vi "StitchTest.vi"() -> ()   [LabVIEW 2014]
uses:
  <vilib>/picture/picture.llb/imagedata.ctl
panel:
  in  "SaveJPEG":bool
  out "Intensity Graph":u8[][](graph)
  out "Yind":i32[](array[numeric])
  out "Xind":i32[](array[numeric])
  out "filenames":string[](array[string])
  in  "PathToVK4":path
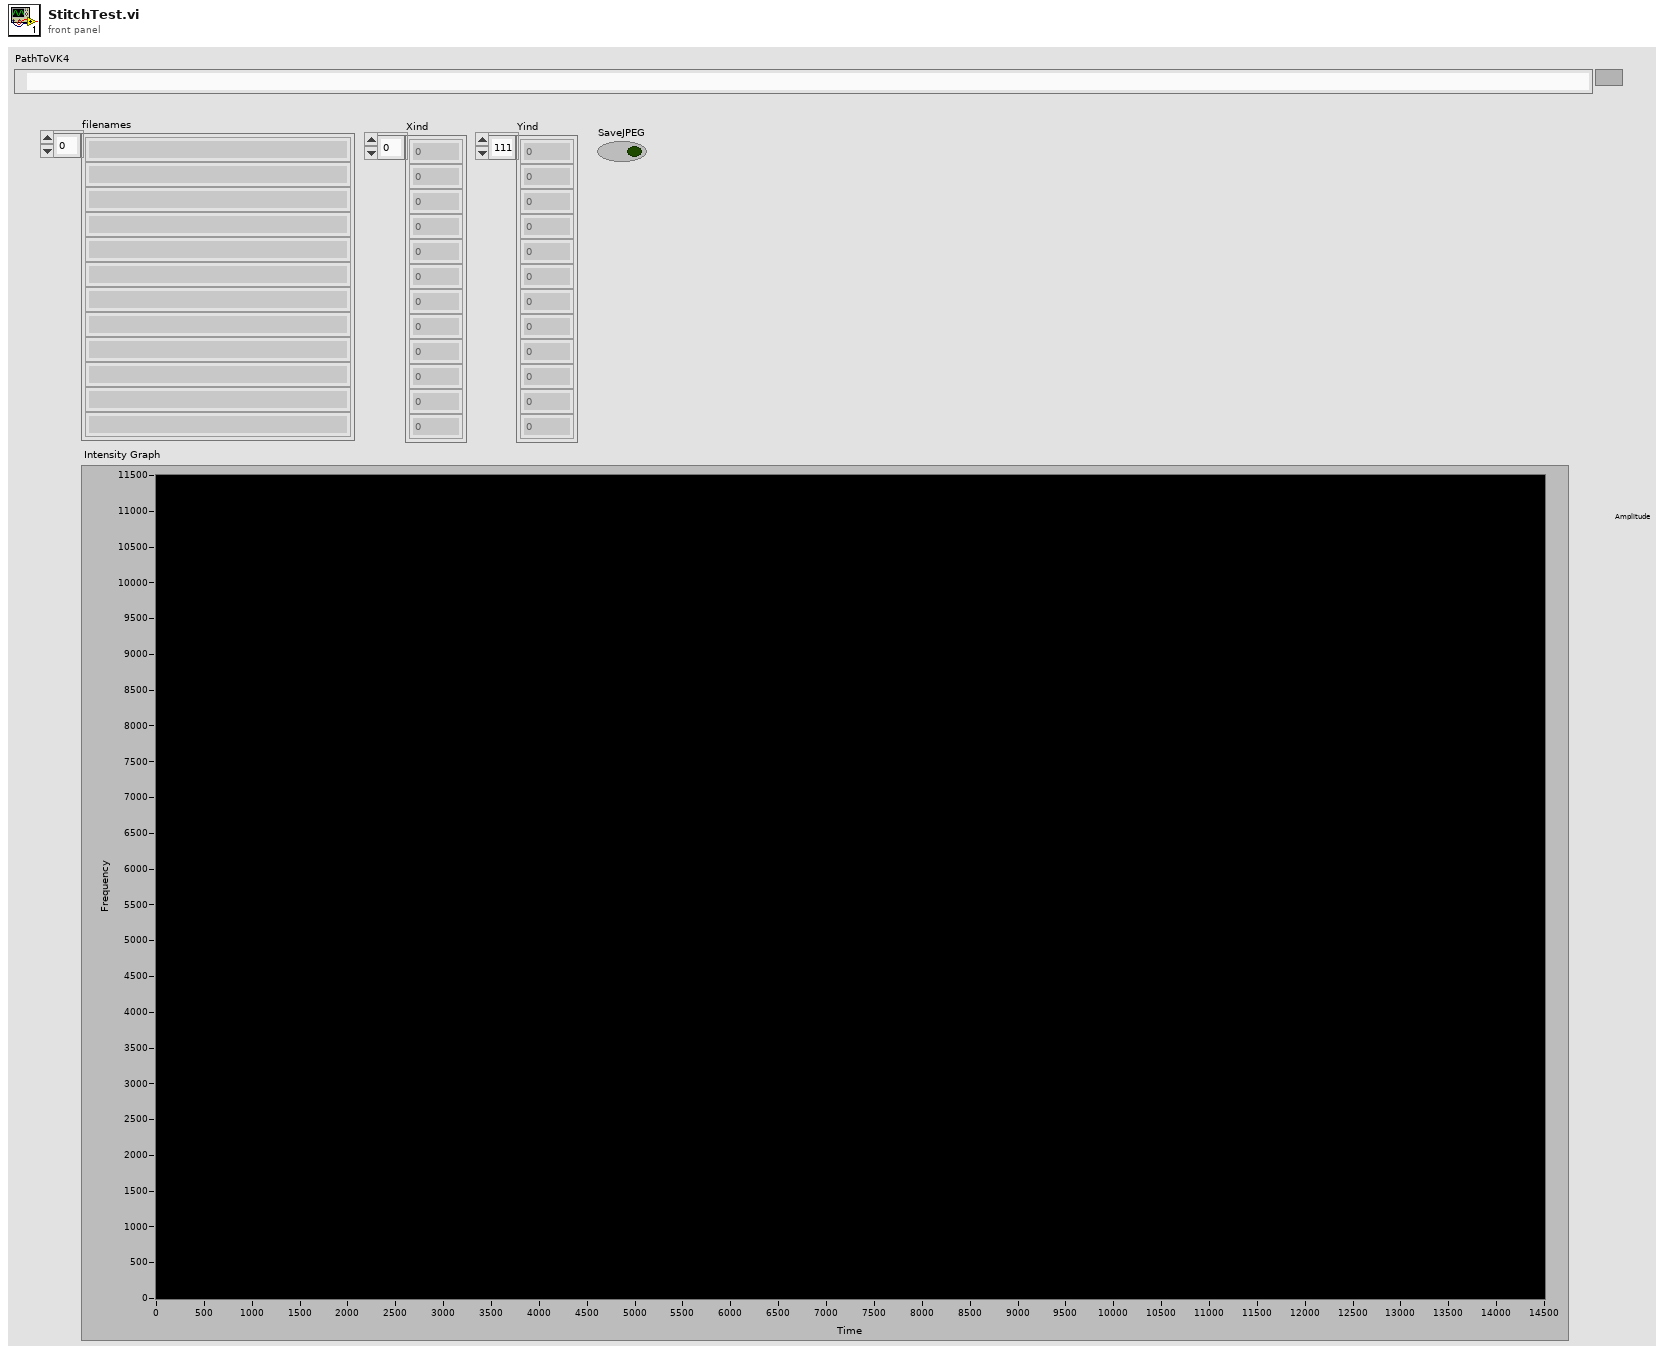
[diagram p1: front panel]
types:
  T1 = cluster{"left":i16, "top":i16, "right":i16, "bottom":i16}
  T2 = typedef "imagedata.ctl" = cluster{"image type":i32, "image depth":i32, "image":u8[], "mask":u8[], "colors":u32[], "Rectangle":cluster{"left":i16, "top":i16, "right":i16, "bottom":i16}}
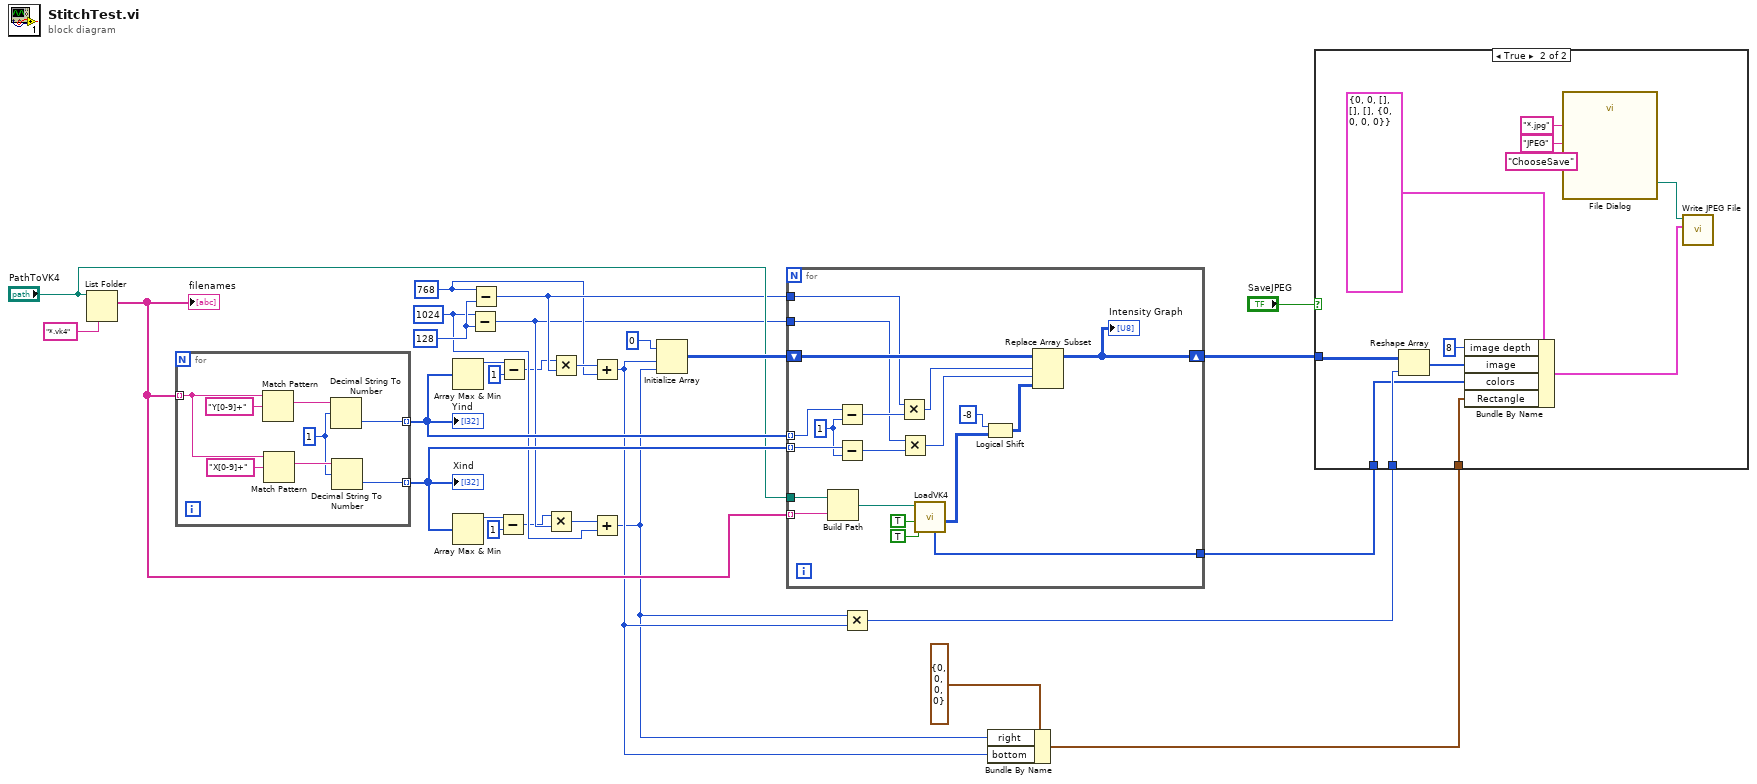
[diagram p0: block diagram]
diagram:
  w17 = 768
  w20 = 128 ("y")
  w16 = 1024
  n1 = List Folder(path="PathToVK4", pattern="*.vk4") -> (filenames=w25:string[])  [unwired: 2 in, 3 out]
  "filenames" <- w25
  n2 = for {
    tunnel: w25 -> [w32] mode=indexing
    tunnel: [w30] -> w23 mode=indexing
    tunnel: [w29] -> w22 mode=indexing
    w31 = 1 ("offset")
    n3 = Match Pattern(string=w32, regular expression="Y[0-9]+") -> (match substring=w35:string)  [unwired: 1 in, 3 out]
    n4 = Match Pattern(string=w32, regular expression="X[0-9]+") -> (match substring=w34:string)  [unwired: 1 in, 3 out]
    n5 = Decimal String To Number(string=w35, offset=w31) -> (number=w30:i32)  [unwired: 1 in, 1 out]
    n6 = Decimal String To Number(string=w34, offset=w31) -> (number=w29:i32)  [unwired: 1 in, 1 out]
  }
  "Xind" <- w22
  "Yind" <- w23
  n7 = Array Max & Min(array=w23) -> (max value=w6:i32)  [unwired: 3 out]
  n8 = Array Max & Min(array=w22) -> (max value=w2:i32)  [unwired: 3 out]
  n9 = Subtract(x=w16, y=w20) -> (x-y=w15:i32)
  n10 = Subtract(x=w17, y=w20) -> (x-y=w18:i32)
  n11 = Subtract(x=w2, y=1) -> (x-y=w1:i32)
  n12 = Subtract(x=w6, y=1) -> (x-y=w5:i32)
  n13 = Multiply(x=w1, y=w15) -> (x*y=w27:i32)
  n14 = Multiply(x=w5, y=w18) -> (x*y=w28:i32)
  n15 = Add(x=w28, y=w17) -> (x+y=w8:i32)
  n16 = Add(x=w27, y=w16) -> (x+y=w7:i32)
  n17 = Initialize Array(u8 0, w8, w7) -> (w24:u8[][])
  n18 = for {
    tunnel: w25 -> [w56] mode=indexing
    tunnel: "PathToVK4" -> [w55]
    tunnel: w23 -> [w51] mode=indexing
    tunnel: w22 -> [w50] mode=indexing
    tunnel: w15 -> [w41]
    shift-right: [w45] -> w14
    shift-left: w24 -> [w46]
    tunnel: w18 -> [w42]
    tunnel: [w37] -> w13
    w49 = 1 ("y")
    n19 = Build Path(base path=w55, name or relative path=w56) -> (appended path=w54:path)
    n20 = Subtract(x=w51, y=w49) -> (x-y=w48:i32)
    n21 = Subtract(x=w50, y=w49) -> (x-y=w47:i32)
    n22 = Multiply(x=w42, y=w48) -> (x*y=w43:i32)
    n23 = Multiply(x=w41, y=w47) -> (x*y=w44:i32)
    n24 = call "LoadVK4.vi"("SaveRaw"=TRUE, "SavePics"=TRUE, "PathToVK4"=w54) -> ("IntenArray"=w40:u16[][], "IntenLU"=w37:u32[])  [unwired: 4 in, 3 out]
    n25 = Logical Shift(y=-8, x=w40) -> (x << y=w38:u16[][])
    n26 = Replace Array Subset(array=w46, new element=w38, index (row)=w43, index (col)=w44) -> (w45:u8[][])
    "Intensity Graph" <- w45
  }
  n27 = Multiply(x=w7, y=w8) -> (x*y=w11:i32)
  n28 = Bundle By Name(cluster=T1 {"left"=0, "top"=0, "right"=0, "bottom"=0} ("Rectangle"), "right"=w7, "bottom"=w8) -> (w9:T1)
  n29 = case shown="True" "SaveJPEG" {
    tunnel: w14 -> [_ w64]
    tunnel: w13 -> [_ w60]
    tunnel: w11 -> [_ w63]
    tunnel: w9 -> [_ w61]
    frame False {
    }
    frame True {
      n30 = Reshape Array(w64, w63) -> (w59:u8[])
      n31 = Bundle By Name(cluster=T2 {"image type"=0, "image depth"=0, "image"=[], "mask"=[], "colors"=[], "Rectangle"={"left"=0, "top"=0, "right"=0, "bottom"=0}} ("image data"), "image depth"=8, "image"=w59, "colors"=w60, "Rectangle"=w61) -> (w57:T2)
      n32 = call "File Dialog"("prompt"="ChooseSave", "pattern (all files)"="*.jpg", "pattern label"="JPEG") -> ("selected path"=w68:path)  [unwired: 9 in, 3 out]
      n33 = call <vilib>:"Write JPEG File.vi"("image data"=w57, "path to JPEG file"=w68) -> ()  [unwired: 8 in, 2 out]
    }
  }
